vi "Teleop.vi"(10 "Match Info":T1={"Autonomous Elapsed Seconds"=0.0, "TeleOp Elapsed Seconds"=0.0, "Disabled Elapsed Seconds"=0.0, "Visited Autonomous"=FALSE, "Visited TeleOp"=FALSE, "Visited Disabled"=FALSE, "Autonomous Settings"={"Autonomous Style"=enum."Independent", "VI Refnum"=refnum}}, 11 "Call Context":T2) -> ()   [LabVIEW 2019]
doc: "This VI is called for each TeleOp packet received from the DS where the robot is not disabled. It is often used to read from the joysticks and update I/O or to update setpoints for timed control loops. It should complete and return within 20 milliseconds or it may miss DS packets."
uses:
  <vilib>/Rock Robotics/WPI/DriverStation/WPI_DriverStationDerivedRobotMode.ctl
  <vilib>/Rock Robotics/WPI/DriverStation/WPI_DriverStationMatch Info.ctl
  <vilib>/Rock Robotics/WPI/Utilities/WPI_GetSetVariantRefNum.vi
  <vilib>/Rock Robotics/Network Tables/NT Write Boolean Array.vi
  <vilib>/Rock Robotics/Network Tables/NT Write Numeric Array.vi
  <vilib>/Rock Robotics/Network Tables/NT Read Boolean.vi
  <vilib>/Rock Robotics/Network Tables/NT Read Number.vi
  <vilib>/Rock Robotics/Network Tables/NT Write Number.vi
panel:
  out "Bottom Limit":bool
  out "Upper Limit":bool
  out "GoDown?":bool
  out "Time":dbl
  out "Throttle":dbl
  out "Sample Slider 0":dbl(slide) scale=0.0..5.0
  out "Sample Boolean 1":bool
  out "Sample Boolean 0":bool
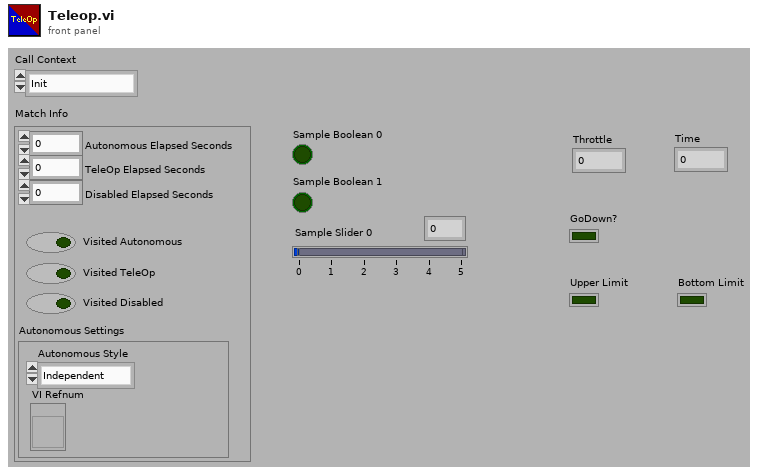
[diagram p1: front panel]
types:
  T1 = typedef "WPI_DriverStationMatch Info.ctl" = cluster{"Autonomous Elapsed Seconds":dbl, "TeleOp Elapsed Seconds":dbl, "Disabled Elapsed Seconds":dbl, "Visited Autonomous":bool, "Visited TeleOp":bool, "Visited Disabled":bool, "Autonomous Settings":cluster{"Autonomous Style":enum16{"Iterative", "Independent"}, "VI Refnum":refnum<vi>}}
  T2 = typedef "WPI_DriverStationDerivedRobotMode.ctl" = enum16{"Init", "Execute", "Stop"}
  T3 = typedef "WPI_RobotDriveDevRef.ctl" = cluster{"DevStatus":errorcluster, "Motors[]":T4[], "Square Inputs":bool, "Max Output":dbl}
  T4 = typedef "WPI_MotorControlDeviceRef.ctl" = cluster{"DeviceStatus":errorcluster, "Type":T5, "PWM":cluster{"PWM Channel":T6, "DeadBand":T7}, "CAN":cluster{"Device Number":u8, "SetOutput VI Ref":variant, "GetOutput VI Ref":variant, "Enable VI Ref":variant, "Disable VI Ref":variant, "Data":variant}, "Invert":bool, "DIO PWM":cluster{"PWM \"Enable\" Channel":T6, "DIOChannel":T8, "PWM Rate":dbl}}
  T5 = typedef "WPI_MotorControlType.ctl" = enum16{"PWM", "CAN", "DIO PWM"}
  T6 = typedef "FPGA_DIOPWMChannel.ctl" = enum8{"PWM 0", "PWM 1", "PWM 2", "PWM 3", "PWM 4", "PWM 5", "PWM 6", "PWM 7", "PWM 8", "PWM 9", "PWM MXP 0", "PWM MXP 1", "PWM MXP 2", "PWM MXP 3", "PWM MXP 4", "PWM MXP 5", "PWM MXP 6", "PWM MXP 7", "PWM MXP 8", "PWM MXP 9", "Invalid"}
  T7 = typedef "WPI_PWMDeadband.ctl" = cluster{"Name":string, "maxPositivePwm":i32, "minPositivePwm":i32, "centerPwm":i32, "maxNegativePwm":i32, "minNegativePwm":i32, "angularRange":u16}
  T8 = typedef "FPGA_DIOChannel.ctl" = enum8{"DIO 0", "DIO 1", "DIO 2", "DIO 3", "DIO 4", "DIO 5", "DIO 6", "DIO 7", "DIO 8", "DIO 9", "DIO MXP 0", "DIO MXP 1", "DIO MXP 2", "DIO MXP 3", "DIO MXP 4", "DIO MXP 5", "DIO MXP 6", "DIO MXP 7", "DIO MXP 8", "DIO MXP 9", "DIO MXP 10", "DIO MXP 11", "DIO MXP 12", "DIO MXP 13", "DIO MXP 14", "DIO MXP 15", "SPI Port CS1", "SPI Port CS2", "SPI Port CS3", "SPI Port MISO", "SPI Port MOSI", "Invalid"}
  T9 = typedef "WPI_JoystickDevRef.ctl" = cluster{"Device":T10}
  T10 = typedef "WPI_JoystickDeviceEnum.ctl" = enum16{"USB 0", "USB 1", "USB 2", "USB 3", "USB 4", "USB 5"}
  T11 = typedef "WPI_SwitchDevRef.ctl" = cluster{"DevStatus":errorcluster, "DIO Channel":T8, "CntIndex":T12, "Normally Closed":bool}
  T12 = typedef "FPGA_CounterCtrSystemIndex.ctl" = enum8{"Ctr 0", "Ctr 1", "Ctr 2", "Ctr 3", "Ctr 4", "Ctr 5", "Ctr 6", "Ctr 7", "Invalid"}
  T13 = typedef "WPI_GyroDevRef.ctl" = cluster{"DevStatus":errorcluster, "Analog Channel":T14, "Gain (VoltsPerDegree/Second)":dbl, "Gyro Type":enum16{"Analog", "XRS450"}, "Handle":i32, "SPI Bus":T15, "Device Found":bool, "Sample Rate":dbl, "Calibrate On Open":bool, "Offset":dbl}
  T14 = typedef "FPGA_AIChannel.ctl" = enum8{"AI 0", "AI 1", "AI 2", "AI 3", "AI MXP 0", "AI MXP 1", "AI MXP 2", "AI MXP 3", "Invalid"}
  T15 = typedef "spi_bus.ctl" = enum16{"SPI On-Board, CS0", "SPI On-Board, CS1", "SPI On-Board, CS2", "SPI On-Board, CS3", "SPI MXP", "Invalid"}
  T16 = typedef "WPI_EncoderDevRef.ctl" = cluster{"DevStatus":errorcluster, "EncoderIndex":T17, "CounterIndex":T12, "DistancePerCount":dbl, "Decoding Type":T18}
  T17 = typedef "FPGA_EncoderIdx.ctl" = enum8{"Enc 0", "Enc 1", "Enc 2", "Enc 3", "Enc 4", "Enc 5", "Enc 6", "Enc 7", "Invalid"}
  T18 = typedef "WPI_EncoderType.ctl" = enum16{"1x", "2x", "4x"}
  T19 = typedef "WPI_AnalogChannelDevRef.ctl" = cluster{"DevStatus":errorcluster, "Analog Channel":T14}
  T20 = typedef "WPI_CompressorDevRef.ctl" = cluster{"DevStatus":errorcluster, "Pneumatics Control Module":u8}
  T21 = typedef "WPI_AccelerometerDevRef.ctl" = cluster{"DevStatus":errorcluster, "Scaling":T22, "Analog Channels":T23, "I2C Bus":T24, "SPI Bus":T15, "Accel Range":T25, "ADXL Axes":T26, "Handle":i32, "Device Address":u8, "Accel Type":enum16{"Analog", "ADXL345 I2C", "ADXL345 SPI", "Internal", "ADXL362 SPI"}}
  T22 = typedef "WPI_AccelerometerScaling.ctl" = cluster{"Gain (VoltsPerG)":dbl, "Center Voltage":dbl}
  T23 = typedef "WPI_AccelerometerAnalogChannels.ctl" = cluster{"X-Axis":T14, "Y-Axis":T14, "Z-Axis":T14}
  T24 = typedef "i2c_bus.ctl" = enum16{"I2C On-Board", "I2C MXP", "Invalid"}
  T25 = typedef "ADXL345 Range.ctl" = u8
  T26 = typedef "WPI_AccelerometerADXL345 Axes.ctl" = cluster{"X-Axis":bool, "Y-Axis":bool, "Z-Axis":bool}
  T27 = cluster{"X-Axis":dbl, "Y-Axis":dbl, "Z-Axis":dbl}
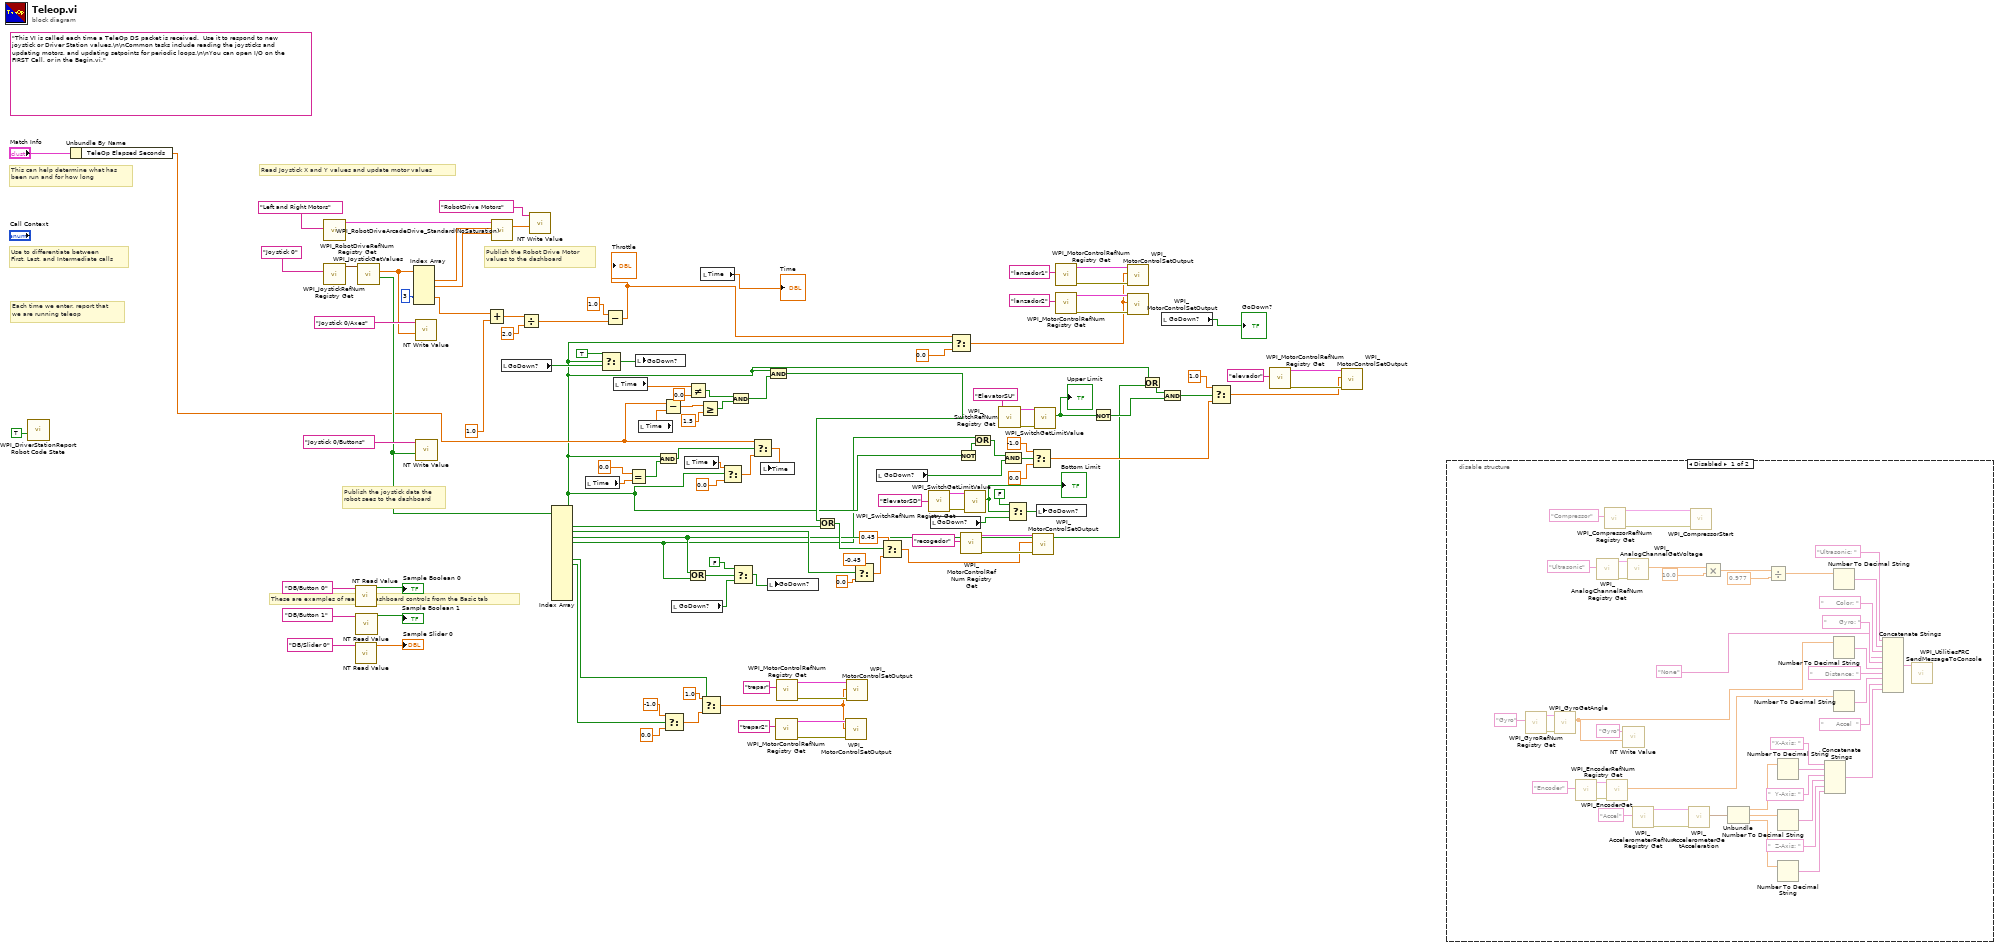
[diagram p0: block diagram]
diagram:
  (unwired) "This VI is called each time a TeleOp DS packet is received.  Use it to respond to new joystick or Driver Station values.\n\nCommon tasks include reading the joysticks and updating motors, and updating setpoints for periodic loops.\n\nYou can open I/O on the FIRST Call, or in the Begin.vi."
  # "These are examples of reading dashboard controls from the Basic tab"
  # "Publish the Robot Drive Motor\nvalues to the dashboard"
  # "Publish the joystick data the\nrobot sees to the dashboard"
  # "Each time we enter, report that\nwe are running teleop"
  # "Use to differentiate between\nFirst, Last, and Intermediate calls"
  # "This can help determine what has\nbeen run and for how long"
  # "Read Joystick X and Y values and update motor values"
  n1 = call <vilib>:"WPI_DriverStationReport Robot Code State.vi"("TeleOp"=TRUE ("Autonomous")) -> ()  [unwired: 10 in, 1 out]
  n2 = Unbundle By Name("Match Info") -> ("TeleOp Elapsed Seconds"=w46:dbl)
  n3 = call <vilib>:"WPI_RobotDriveRefNum Registry Get.vi"("refnum name"="Left and Right Motors") -> ("RobotDriveDevRef"=w114:T3)  [unwired: 1 in, 9 out]
  n4 = call <vilib>:"WPI_JoystickRefNum Registry Get.vi"("refnum name"="Joystick 0") -> ("JoystickDevRef"=w111:T9)  [unwired: 1 in, 9 out]
  n5 = call-poly <vilib>:"NT Read Value.vi"("Name"="DB/Button 0" ("refnum name")) -> ("Boolean"=→"Sample Boolean 0":bool)  [unwired: 9 in, 1 out]
  n6 = call-poly <vilib>:"NT Read Value.vi"("Name"="DB/Slider 0" ("refnum name")) -> ("Numeric"=→"Sample Slider 0":dbl)  [unwired: 9 in, 1 out]
  n7 = call-poly <vilib>:"NT Read Value.vi"("Name"="DB/Button 1" ("refnum name")) -> ("Boolean"=→"Sample Boolean 1":bool)  [unwired: 9 in, 1 out]
  n8 = call <vilib>:"WPI_JoystickGetValues.vi"("JoystickDevRef"=w111) -> ("Buttons"=w98:bool[], "Axes"=w107:dbl[])  [unwired: 6 in, 3 out]
  n9 = Index Array(array=w107, index #4=3 ("index")) -> (element #1=w113:dbl, element #2=w14:dbl, element #4=w13:dbl)  [unwired: 4 in, 2 out]
  n10 = call-poly <vilib>:"NT Write Value.vi"("Numeric Array"=w107, "Name"="Joystick 0/Axes") -> ()  [unwired: 9 in, 1 out]
  n11 = call-poly <vilib>:"NT Write Value.vi"("Boolean Array"=w98, "Name"="Joystick 0/Buttons") -> ()  [unwired: 9 in, 1 out]
  n12 = Add(x=w13, y=1.0) -> (x+y=w77:dbl)
  n13 = call <vilib>:"WPI_RobotDriveArcadeDrive_Standard(NoSaturation).vi"("Y axis value"=w14, "X axis value"=w113, "RobotDriveDevRef"=w114) -> ("Motor Values"=w100:dbl[])  [unwired: 1 in, 7 out]
  n14 = local read "GoDown?"() -> (w28:bool)
  n15 = Divide(x=w77, y=2.0) -> (x/y=w75:dbl)
  n16 = call-poly <vilib>:"NT Write Value.vi"("Numeric Array"=w100, "Name"="RobotDrive Motors") -> ()  [unwired: 9 in, 1 out]
  n17 = Index Array(array=w98) -> (element #1=w11:bool, element #2=w34:bool, element #3=w96:bool, element #4=w6:bool, element #5=w5:bool, element #8=w82:bool, element #9=w81:bool)  [unwired: 15 in, 8 out]
  n18 = local read "Time"() -> (w63:dbl)
  n19 = Select(t=TRUE, s=w11, f=w28) -> (s? t:f=w29:bool)
  n20 = Subtract(x=1.0, y=w75) -> (x-y=w12:dbl)
  "Throttle" <- w12
  n21 = local read "Time"() -> (w40:dbl)
  n22 = Equal?(x=0.0, y=w63) -> (x = y?=w64:bool)
  n23 = local write "GoDown?"(w29) -> ()
  n24 = local read "Time"() -> (w45:dbl)
  n25 = And(x=w11, y=w64) -> (x .and. y?=w65:bool)
  n26 = Subtract(x=w46, y=w45) -> (x-y=w44:dbl)
  n27 = Select(t=-1.0, s=w81, f=0.0) -> (s? t:f=w88:dbl)
  n28 = local read "GoDown?"() -> (w2:bool)
  n29 = local read "Time"() -> (w37:dbl)
  n30 = Not Equal?(x=w40, y=0.0) -> (x != y?=w41:bool)
  n31 = Or(x=w6, y=w5) -> (x .or. y?=w4:bool)
  n32 = Greater Or Equal?(x=w44, y=1.5) -> (x >= y?=w42:bool)
  n33 = Select(t=1.0, s=w82, f=w88) -> (s? t:f=w17:dbl)
  n34 = local read "Time"() -> (→"Time":dbl)
  n35 = Select(t=w37, s=w11, f=0.0) -> (s? t:f=w35:dbl)
  n36 = And(x=w41, y=w42) -> (x .and. y?=w38:bool)
  n37 = Select(t=FALSE, s=w4, f=w2) -> (s? t:f=w3:bool)
  n38 = Select(t=w46, s=w65, f=w35) -> (s? t:f=w66:dbl)
  n39 = local write "Time"(w66) -> ()
  n40 = And(x=w11, y=w38) -> (x .and. y?=w32:bool)
  n41 = local write "GoDown?"(w3) -> ()
  n42 = call <vilib>:"WPI_MotorControlRefNum Registry Get.vi"("refnum name"="trepar2") -> ("error out"=w20:errorcluster, "MotorControlDevRef"=w19:T4)  [unwired: 9 in]
  n43 = call <vilib>:"WPI_MotorControlRefNum Registry Get.vi"("refnum name"="trepar") -> ("error out"=w86:errorcluster, "MotorControlDevRef"=w84:T4)  [unwired: 9 in]
  n44 = Or(x=w32, y=w34) -> (x .or. y?=w33:bool)
  n45 = call <vilib>:"WPI_MotorControlSetOutput.vi"("error in (no error)"=w20, "Output"=w17, "MotorControlDevRef"=w19) -> ()  [unwired: 6 in, 3 out]
  n46 = call <vilib>:"WPI_MotorControlSetOutput.vi"("error in (no error)"=w86, "Output"=w17, "MotorControlDevRef"=w84) -> ()  [unwired: 6 in, 3 out]
  n47 = Select(t=-0.45, s=w96, f=0.0) -> (s? t:f=w93:dbl)
  n48 = local read "GoDown?"() -> (w24:bool)
  n49 = Select(t=0.45, s=w33, f=w93) -> (s? t:f=w89:dbl)
  n50 = call <vilib>:"WPI_SwitchRefNum Registry Get.vi"("refnum name"="ElevatorSD") -> ("error out"=w51:errorcluster, "SwitchDevRef"=w52:T11)  [unwired: 9 in]
  n51 = local read "GoDown?"() -> (w26:bool)
  n52 = Select(t=w12, s=w11, f=0.0) -> (s? t:f=w61:dbl)
  n53 = Not(x=w11) -> (.not. x?=w9:bool)
  n54 = call <vilib>:"WPI_MotorControlRefNum Registry Get.vi"("refnum name"="recogedor") -> ("error out"=w90:errorcluster, "MotorControlDevRef"=w92:T4)  [unwired: 9 in]
  n55 = call <vilib>:"WPI_SwitchGetLimitValue.vi"("error in (no error)"=w51, "SwitchDevRef"=w52) -> ("Switch Pressed"=w21:bool)  [unwired: 7 in, 2 out]
  "Bottom Limit" <- w21
  n56 = Or(x=w5, y=w9) -> (x .or. y?=w8:bool)
  n57 = call <vilib>:"WPI_SwitchRefNum Registry Get.vi"("refnum name"="ElevatorSU") -> ("error out"=w58:errorcluster, "SwitchDevRef"=w59:T11)  [unwired: 9 in]
  n58 = And(x=w8, y=w24) -> (x .and. y?=w31:bool)
  n59 = Select(t=FALSE, s=w21, f=w26) -> (s? t:f=w25:bool)
  n60 = Select(t=-1.0, s=w31, f=0.0) -> (s? t:f=w7:dbl)
  n61 = call <vilib>:"WPI_MotorControlSetOutput.vi"("error in (no error)"=w90, "Output"=w89, "MotorControlDevRef"=w92) -> ()  [unwired: 6 in, 3 out]
  n62 = call <vilib>:"WPI_SwitchGetLimitValue.vi"("error in (no error)"=w58, "SwitchDevRef"=w59) -> ("Switch Pressed"=w22:bool)  [unwired: 7 in, 2 out]
  "Upper Limit" <- w22
  n63 = local write "GoDown?"(w25) -> ()
  n64 = call <vilib>:"WPI_MotorControlRefNum Registry Get.vi"("refnum name"="lanzador1") -> ("error out"=w68:errorcluster, "MotorControlDevRef"=w70:T4)  [unwired: 9 in]
  n65 = call <vilib>:"WPI_MotorControlRefNum Registry Get.vi"("refnum name"="lanzador2") -> ("error out"=w71:errorcluster, "MotorControlDevRef"=w73:T4)  [unwired: 9 in]
  n66 = Not(x=w22) -> (.not. x?=w49:bool)
  n67 = call <vilib>:"WPI_MotorControlSetOutput.vi"("error in (no error)"=w68, "Output"=w61, "MotorControlDevRef"=w70) -> ()  [unwired: 6 in, 3 out]
  n68 = call <vilib>:"WPI_MotorControlSetOutput.vi"("error in (no error)"=w71, "Output"=w61, "MotorControlDevRef"=w73) -> ()  [unwired: 6 in, 3 out]
  n69 = Or(x=w11, y=w6) -> (x .or. y?=w10:bool)
  n70 = local read "GoDown?"() -> (→"GoDown?":bool)
  n71 = And(x=w10, y=w49) -> (x .and. y?=w56:bool)
  n72 = Select(t=1.0, s=w56, f=w7) -> (s? t:f=w23:dbl)
  n73 = call <vilib>:"WPI_MotorControlRefNum Registry Get.vi"("refnum name"="elevador") -> ("error out"=w53:errorcluster, "MotorControlDevRef"=w55:T4)  [unwired: 9 in]
  n74 = call <vilib>:"WPI_MotorControlSetOutput.vi"("error in (no error)"=w53, "Output"=w23, "MotorControlDevRef"=w55) -> ()  [unwired: 6 in, 3 out]
  n75 = disable-structure shown="Disabled" {
    frame Disabled {
      n76 = call <vilib>:"WPI_GyroRefNum Registry Get.vi"("refnum name"="Gyro") -> ("error out"=w147:errorcluster, "GyroDevRef"=w148:T13)  [unwired: 9 in]
      n77 = call <vilib>:"WPI_GyroGetAngle.vi"("error in"=w147, "GyroDevRef"=w148) -> ("Angle"=w121:dbl)  [unwired: 5 in, 4 out]
      n78 = call <vilib>:"WPI_EncoderRefNum Registry Get.vi"("refnum name"="Encoder") -> ("error out"=w142:errorcluster, "EncoderDevRef"=w143:T16)  [unwired: 9 in]
      n79 = call <vilib>:"WPI_AnalogChannelRefNum Registry Get.vi"("refnum name"="Ultrasonic") -> ("error out"=w159:errorcluster, "AIDeviceRef"=w160:T19)  [unwired: 9 in]
      n80 = call <vilib>:"WPI_CompressorRefNum Registry Get.vi"("refnum name"="Compressor") -> ("error out"=w119:errorcluster, "CompressorDevRef"=w120:T20)  [unwired: 9 in]
      n81 = call <vilib>:"WPI_EncoderGet.vi"("error in (no error)"=w142, "EncoderDevRef"=w143) -> ("Distance"=w140:dbl)  [unwired: 4 in, 5 out]
      n82 = call-poly <vilib>:"NT Write Value.vi"("Numeric"=w121, "Name"="Gyro") -> ()  [unwired: 9 in, 1 out]
      n83 = call <vilib>:"WPI_AnalogChannelGetVoltage.vi"("error in (no error)"=w159, "AIDeviceRef"=w160) -> ("Voltage"=w157:dbl)  [unwired: 7 in, 2 out]
      n84 = call <vilib>:"WPI_AccelerometerRefNum Registry Get.vi"("refnum name"="Accel") -> ("error out"=w135:errorcluster, "AccelerometerDevRef"=w136:T21)  [unwired: 9 in]
      n85 = call <vilib>:"WPI_AccelerometerGetAcceleration.vi"("error in"=w135, "AccelerometerDevRef"=w136) -> ("Accelerations"=w134:T27)  [unwired: 7 in, 2 out]
      n86 = call <vilib>:"WPI_CompressorStart.vi"("error in (no error)"=w119, "CompressorDevRef"=w120) -> ()  [unwired: 8 in, 2 out]
      n87 = Multiply(x=w157, y=10.0) -> (x*y=w155:dbl)
      n88 = Unbundle(w134) -> ("X-Axis"=w131:dbl, "Y-Axis"=w129:dbl, "Z-Axis"=w128:dbl)
      n89 = Divide(x=w155, y=0.977) -> (x/y=w153:dbl)
      n90 = Number To Decimal String(number=w131) -> (decimal integer string=w130:string)  [unwired: 1 in]
      n91 = Number To Decimal String(number=w129) -> (decimal integer string=w127:string)  [unwired: 1 in]
      n92 = Number To Decimal String(number=w128) -> (decimal integer string=w126:string)  [unwired: 1 in]
      n93 = Concatenate Strings("X-Axis: " ("string"), w130, "  Y-Axis: " ("string"), w127, "  Z-Axis: " ("string"), w126) -> (w123:string)
      n94 = Number To Decimal String(number=w153) -> (decimal integer string=w151:string)  [unwired: 1 in]
      n95 = Number To Decimal String(number=w121) -> (decimal integer string=w145:string)  [unwired: 1 in]
      n96 = Number To Decimal String(number=w140) -> (decimal integer string=w138:string)  [unwired: 1 in]
      n97 = Concatenate Strings("Ultrasonic: " ("string"), w151, "      Color: " ("string"), "None" ("string"), "      Gyro: " ("string"), w145, "      Distance: " ("string"), w138, "      Accel  " ("string"), w123) -> (w144:string)
      n98 = call <vilib>:"WPI_UtilitiesFRC SendMessageToConsole.vi"("Message"=w144) -> ()  [unwired: 14 in, 1 out]
    }
    frame Enabled {
    }
  }
